vi "SaveDataTDCV775.vi"(6 "Module":string="TDC", 8 "error in (no error)":errorcluster, 9 "Buff":u32[](array[numeric]), 10 "File Handle":T1 format="%.0x", 11 "String":string) -> (0 "error out":errorcluster, 3 "# Events Acquired (VME)":u32)   [LabVIEW 2014]
uses:
  <vilib>/addons/h5labview2/base/hid_t.ctl
  <vilib>/addons/h5labview2/base/lib_path.vi
  <vilib>/addons/h5labview2/base/H5Equery.vi
  <vilib>/addons/h5labview2/dataset/H5Dwrite.llb/H5Dwrite.xnode
  <vilib>/addons/h5labview2/group/H5G.lvlib
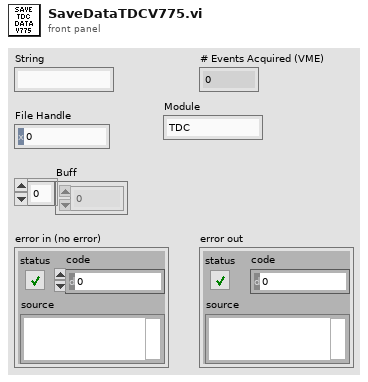
[diagram p1: front panel]
types:
  T1 = typedef "hid_t.ctl" = i32
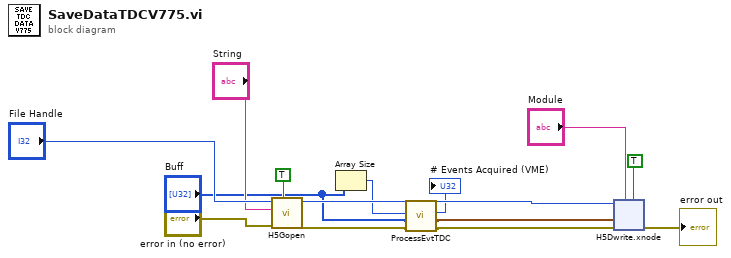
[diagram p0: block diagram]
diagram:
  n1 = call <vilib>:"H5Gopen.vi"("create? (F)"=TRUE, "error in (no error)"="error in (no error)", "name"="String", "ref in"="File Handle") -> ("error out"=w6:errorcluster, "group out"=w12:T1)  [unwired: 6 in]
  n2 = Array Size(array="Buff") -> (size(s)=w4:i32)
  n3 = call "ProcessEvtTDC.vi"("error in"=w6, "Encoded Data"="Buff", "# data points in evt"=w4) -> ("error out"=w2:errorcluster, "Decoded Data"=w3:cluster{"Channel":u8, "TDC Data":u16}[], "# Events"=→"# Events Acquired (VME)":u32)  [unwired: 6 in]
  n4 = xnode "H5Dwrite.xnode"("replace? (F)"=TRUE, "dataset name"="Module", "error in (no error)"=w2, "data"=w3, "ref in"=w12) -> ("error out"=→"error out":errorcluster)  [unwired: 2 in, 2 out]
